vi "Write Intensity Graph ref.vi"(8 "error in (no error)":errorcluster, 9 "Intensity Graph (Control)":refnum<vi>, 10 "Intensity Graph":refnum<vi>, 11 "graph_utilities in":refnum<class "graph_utilities.lvclass">) -> (0 "error out":errorcluster, 3 "graph_utilities out":refnum<class "graph_utilities.lvclass">)   [LabVIEW 2019, in "graph_utilities.lvclass"]
doc: "Write Intensity Graph control references to the class wire.\n- \"Intensity Graph\" is the normal target for reading and writing.\n- \"Intensity Graph (Control)\" is only used to read the cursor position of the \"Control\" Intensity Graph."
uses:
  graph_utilities.lvclass
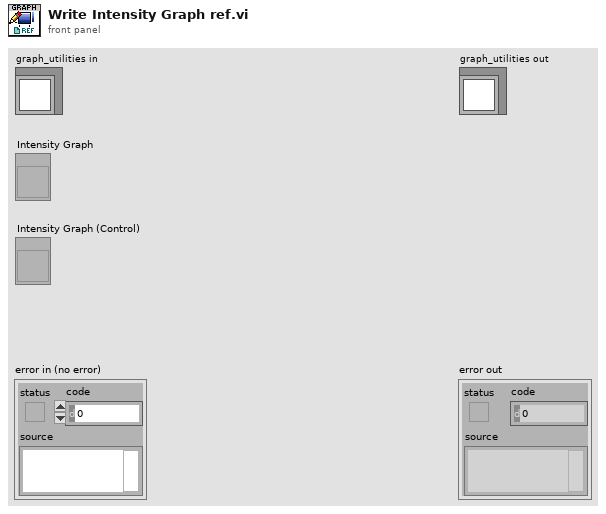
[diagram p1: front panel]
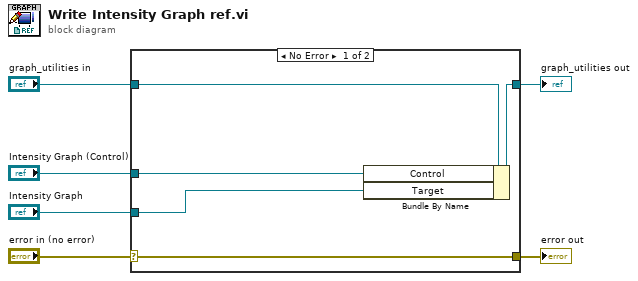
[diagram p0: block diagram]
diagram:
  n1 = case shown="No Error" "error in (no error)" {
    selector: "error in (no error)" -> [w11 w12]
    tunnel: [w11 w12] -> w5
    tunnel: [w9 w13] -> w3
    tunnel: "graph_utilities in" -> [w10 w13]
    tunnel: "Intensity Graph (Control)" -> [w8 _]
    tunnel: "Intensity Graph" -> [w7 _]
    frame No Error {
      n2 = Bundle By Name(cluster=w10, "Control"=w8, "Target"=w7) -> (w9:refnum<class "graph_utilities.lvclass">)
    }
    frame Error {
    }
  }
  "error out" <- w5
  "graph_utilities out" <- w3
